vi "Generate Report.vi"(8 "error in (no error)":errorcluster, 10 "Resource In":variant, 11 "HIJ Vision File Viewer in":refnum<class "HIJ Vision File Viewer.lvclass">) -> (0 "error out":errorcluster, 2 "Resource Out":variant, 3 "HIJ Vision File Viewer out":refnum<class "HIJ Vision File Viewer.lvclass">)   [LabVIEW 2014, in "HIJ Vision File Viewer.lvlib" / "HIJ Vision File Viewer.lvclass"]
uses:
  HIJ Vision File Viewer.lvclass
  HIJ Vision Display/HIJ Vision Display/HIJ Vision Display.lvclass/HIJ Vision Display.ctl
  HIJ Vision Display/HIJ Vision Display/Write Save Report_.vi
  HIJ Vision Display/HIJ Vision Display/HIJ Vision Display.lvclass
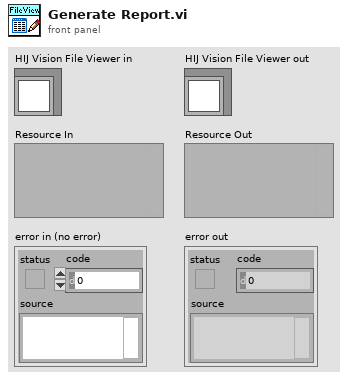
[diagram p1: front panel]
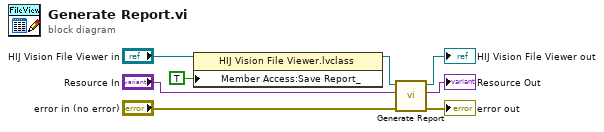
[diagram p0: block diagram]
diagram:
  n1 = property class="HIJ Vision File Viewer.lvclass"(reference="HIJ Vision File Viewer in", "Member Access:Save Report_"=TRUE ("Save Report_")) -> (reference out=w2:refnum<class "HIJ Vision File Viewer.lvclass">)  [unwired: 1 in, 1 out]
  n2 = call-parent "Generate Report.vi"("error in (no error)"="error in (no error)", "Resource In"="Resource In", "HIJ Vision Display in"=w2) -> ("error out"=→"error out":errorcluster, "Resource Out"=→"Resource Out":variant, "HIJ Vision Display out"=→"HIJ Vision File Viewer out":refnum<class "HIJ Vision File Viewer.lvclass">)  [unwired: 6 in]
